vi "Tab_constant.vi"() -> ()   [LabVIEW 2017]
panel:
  in  "Outer Tab":enum32{"Page 1", "Page 2"}(tab)
  in  "Inner Tab":enum32{"Page 1", "Page 2"}(tab)
  in  "Numeric":dbl
  in  "Array":dbl[](array[numeric])
  in  "Enum":enum16{"Apple", "Oranges", "Pears"}(ring)
  in  "String":string
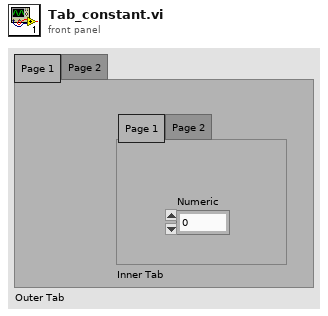
[diagram p1: front panel]
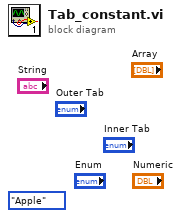
[diagram p0: block diagram]
diagram:
  (unwired) enum16{"Apple", "Oranges", "Pears"}."Apple" ("Enum")
